vi "1D sweep iteration instruction generator (SubVI).vi"(6 "Maximum value B [µT]":dbl, 7 "Minimum value B [µT]":dbl, 9 "Number of steps":dbl, 10 "Current iteration":i32, 11 "Direction field sweep":string) -> (3 "Current [µT]":dbl, 4 "Magnetic field strength":dbl, 5 "String":string)   [LabVIEW 2018]
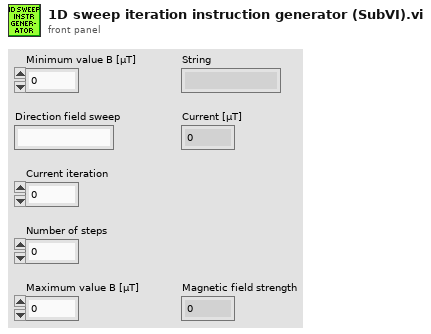
[diagram p1: front panel]
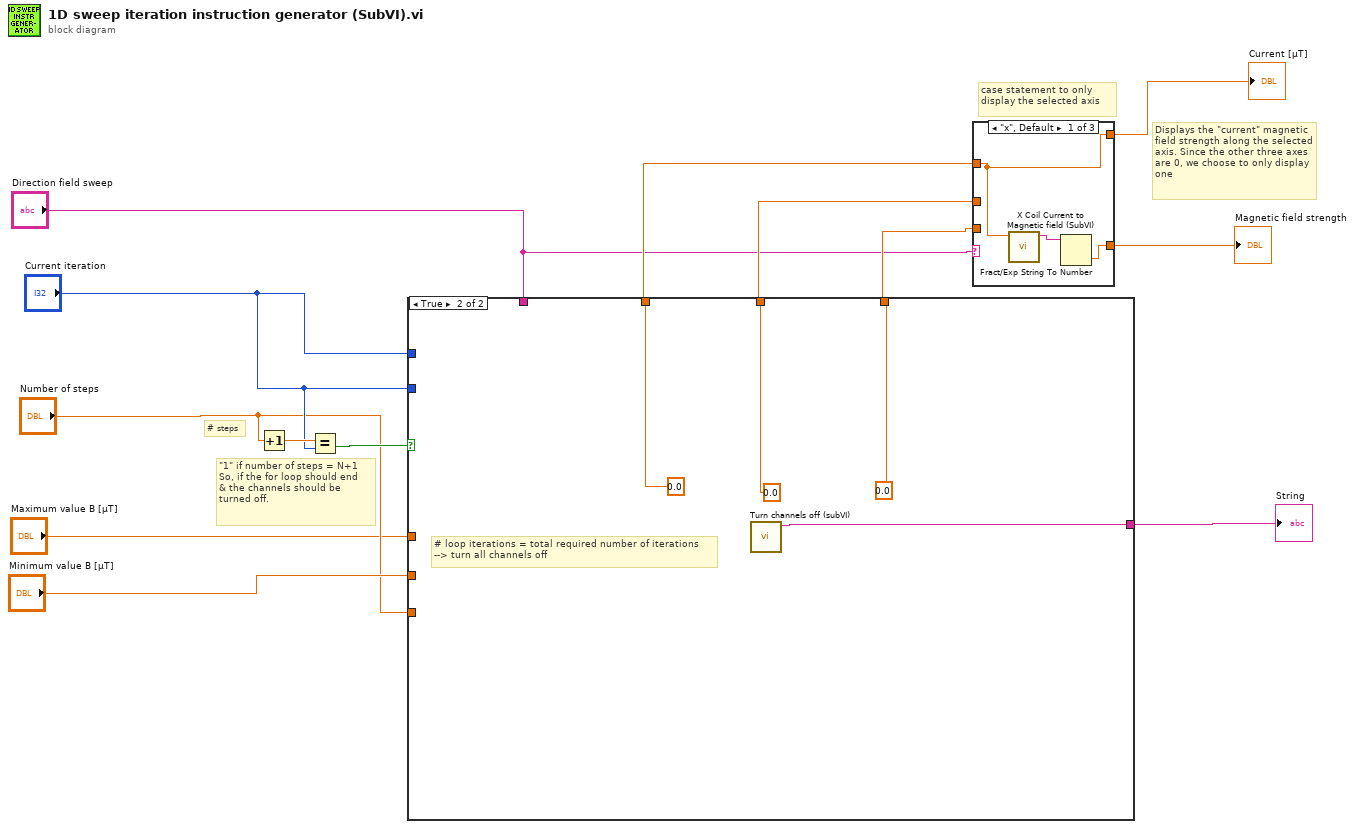
[diagram p0: block diagram]
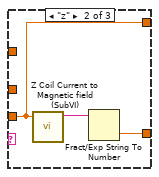
[diagram p2: hidden frame]
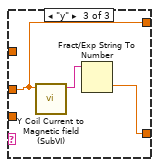
[diagram p3: hidden frame]
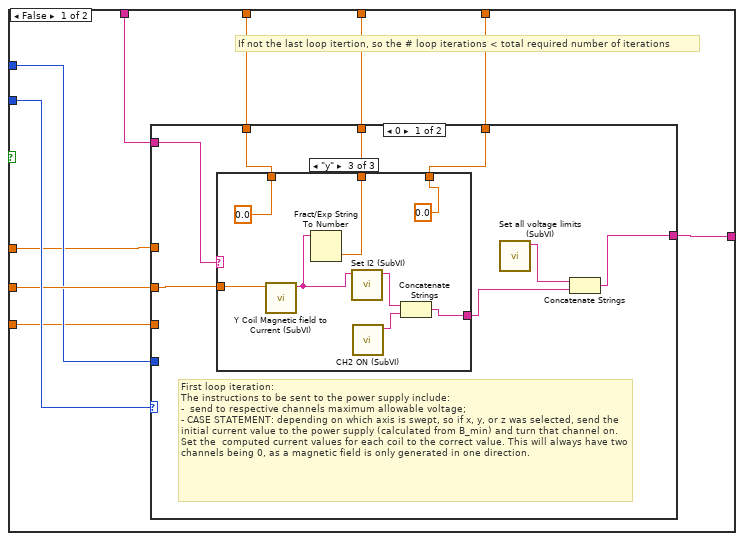
[diagram p4: hidden frame]
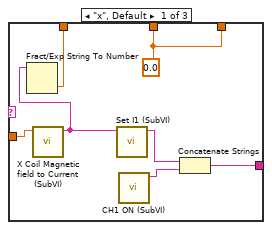
[diagram p5: hidden frame]
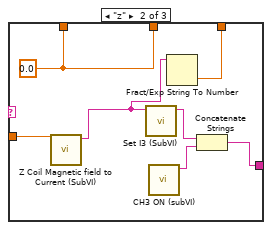
[diagram p6: hidden frame]
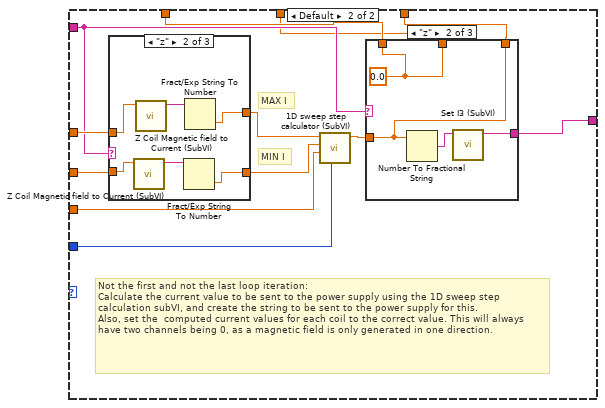
[diagram p7: hidden frame]
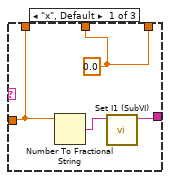
[diagram p8: hidden frame]
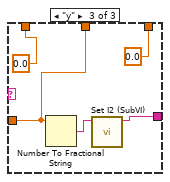
[diagram p9: hidden frame]
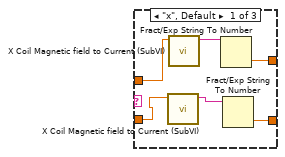
[diagram p10: hidden frame]
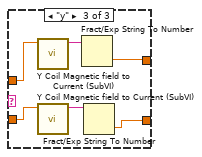
[diagram p11: hidden frame]
diagram:
  # "case statement to only display the selected axis"
  # "Displays the \"current\" magnetic field strength along the selected axis. Since the other three axes are 0, we choose to only display  one"
  # "\"1\" if number of steps = N+1\nSo, if the for loop should end \n& the channels should be \nturned off."
  # "# steps"
  n1 = Increment(x="Number of steps") -> (x+1=w8:dbl)
  n2 = Equal?(x=w8, y="Current iteration") -> (x = y?=w4:bool)
  n3 = case shown="True" w4 {
    tunnel: [w15 0.0 ("Magnetic field x [µT]")] -> w10
    tunnel: [w17 0.0 ("Magnetic field y [µT]")] -> w11
    tunnel: [w16 0.0 ("Magnetic field z [µT]")] -> w12
    tunnel: "Current iteration" -> [w23 _]
    tunnel: "Direction field sweep" -> [w22 _]
    tunnel: "Minimum value B [µT]" -> [w21 _]
    tunnel: "Current iteration" -> [w20 _]
    tunnel: "Number of steps" -> [w19 _]
    tunnel: "Maximum value B [µT]" -> [w18 _]
    tunnel: [w14 w97] -> w6
    frame False {
      # "If not the last loop itertion, so the # loop iterations < total required number of iterations"
      n4 = case shown="0" w23 {
        tunnel: w22 -> [w30 w59]
        tunnel: w21 -> [w31 w65]
        tunnel: w20 -> [_ w60]
        tunnel: w19 -> [_ w61]
        tunnel: w18 -> [_ w64]
        tunnel: [w26 w56] -> w15
        tunnel: [w25 w54] -> w17
        tunnel: [w24 w55] -> w16
        tunnel: [w27 w58] -> w14
        frame 0 {
          # "First loop iteration: \nThe instructions to be sent to the power supply include:\n-  send to respective channels maximum allowable voltage;\n- CASE STATEMENT: depending on which axis is swept, so if x, y, or z was selected, send the initial current value to the power supply (calculated from B_min) and turn that channel on.\nSet the  computed current values for each coil to the correct value. This will always have two channels being 0, as a magnetic field is only generated in one direction."
          n5 = case shown="\"y\"" w30 {
            tunnel: w31 -> [w38 w45 w53]
            tunnel: [w35 w44 w48] -> w29
            tunnel: [w33 w41 0.0 ("Magnetic field y [µT]")] -> w26
            tunnel: [w32 w41 w52] -> w25
            tunnel: [w32 w40 0.0 ("Magnetic field y [µT]")] -> w24
            frame "x", Default {
              w32 = 0.0 ("Magnetic field y [µT]")
              n6 = call "X Coil Magnetic field to Current (SubVI).vi"("Magnetic field [µT]"=w38) -> ("Current X"=w34:string)  [unwired: 10 in]
              n7 = Fract/Exp String To Number(string=w34) -> (number=w33:dbl)  [unwired: 3 in, 1 out]
              n8 = call "Set I1 (SubVI).vi"("Current X"=w34) -> ("String instruction"=w36:string)  [unwired: 10 in]
              n9 = call "CH1 ON (SubVI).vi"() -> ("String"=w37:string)  [unwired: 11 in]
              n10 = Concatenate Strings(w36, w37) -> (w35:string)
            }
            frame "z" {
              w41 = 0.0 ("Magnetic field y [µT]")
              n11 = call "Z Coil Magnetic field to Current (SubVI).vi"("Magnetic field [µT]"=w45) -> ("Current Z"=w39:string)  [unwired: 10 in]
              n12 = call "Set I3 (SubVI).vi"("Current Z"=w39) -> ("String"=w43:string)  [unwired: 10 in]
              n13 = call "CH3 ON (subVI).vi"() -> ("String"=w42:string)  [unwired: 11 in]
              n14 = Fract/Exp String To Number(string=w39) -> (number=w40:dbl)  [unwired: 3 in, 1 out]
              n15 = Concatenate Strings(w43, w42) -> (w44:string)
            }
            frame "y" {
              n16 = call "Y Coil Magnetic field to Current (SubVI).vi"("Magnetic field [µT]"=w53) -> ("Current Y"=w51:string)  [unwired: 10 in]
              n17 = Fract/Exp String To Number(string=w51) -> (number=w52:dbl)  [unwired: 3 in, 1 out]
              n18 = call "Set I2 (SubVI).vi"("Current Y"=w51) -> ("String"=w49:string)  [unwired: 10 in]
              n19 = call "CH2 ON (SubVI).vi"() -> ("String"=w50:string)  [unwired: 11 in]
              n20 = Concatenate Strings(w49, w50) -> (w48:string)
            }
          }
          n21 = call "Set all voltage limits (SubVI).vi"() -> ("String"=w28:string)  [unwired: 11 in]
          n22 = Concatenate Strings(w28, w29) -> (w27:string)
        }
        frame Default {
          # "Not the first and not the last loop iteration: \nCalculate the current value to be sent to the power supply using the 1D sweep step calculation subVI, and create the string to be sent to the power supply for this.  \nAlso, set the  computed current values for each coil to the correct value. This will always have two channels being 0, as a magnetic field is only generated in one direction."
          # "MIN I"
          # "MAX I"
          n23 = case shown="\"z\"" w59 {
            tunnel: w65 -> [w84 w90 w96]
            tunnel: w64 -> [w83 w87 w93]
            tunnel: [w80 w85 w91] -> w63
            tunnel: [w79 w88 w94] -> w62
            frame "x", Default {
              n24 = call "X Coil Magnetic field to Current (SubVI).vi"("Magnetic field [µT]"=w84) -> ("Current X"=w81:string)  [unwired: 10 in]
              n25 = call "X Coil Magnetic field to Current (SubVI).vi"("Magnetic field [µT]"=w83) -> ("Current X"=w82:string)  [unwired: 10 in]
              n26 = Fract/Exp String To Number(string=w82) -> (number=w80:dbl)  [unwired: 3 in, 1 out]
              n27 = Fract/Exp String To Number(string=w81) -> (number=w79:dbl)  [unwired: 3 in, 1 out]
            }
            frame "z" {
              n28 = call "Z Coil Magnetic field to Current (SubVI).vi"("Magnetic field [µT]"=w90) -> ("Current Z"=w89:string)  [unwired: 10 in]
              n29 = call "Z Coil Magnetic field to Current (SubVI).vi"("Magnetic field [µT]"=w87) -> ("Current Z"=w86:string)  [unwired: 10 in]
              n30 = Fract/Exp String To Number(string=w89) -> (number=w88:dbl)  [unwired: 3 in, 1 out]
              n31 = Fract/Exp String To Number(string=w86) -> (number=w85:dbl)  [unwired: 3 in, 1 out]
            }
            frame "y" {
              n32 = call "Y Coil Magnetic field to Current (SubVI).vi"("Magnetic field [µT]"=w93) -> ("Current Y"=w92:string)  [unwired: 10 in]
              n33 = call "Y Coil Magnetic field to Current (SubVI).vi"("Magnetic field [µT]"=w96) -> ("Current Y"=w95:string)  [unwired: 10 in]
              n34 = Fract/Exp String To Number(string=w92) -> (number=w91:dbl)  [unwired: 3 in, 1 out]
              n35 = Fract/Exp String To Number(string=w95) -> (number=w94:dbl)  [unwired: 3 in, 1 out]
            }
          }
          n36 = call "1D sweep step calculator (SubVI).vi"("Iteration"=w60, "Number of steps"=w61, "Minimum current"=w62, "Maximum current"=w63) -> ("Current at this iteration"=w57:dbl)  [unwired: 7 in]
          n37 = case shown="\"z\"" w59 {
            tunnel: [w69 w73 w78] -> w58
            tunnel: w57 -> [w66 w70 w74]
            tunnel: [w66 w72 0.0 ("Magnetic field y [µT]")] -> w56
            tunnel: [w68 w70 0.0 ("Magnetic field y [µT]")] -> w55
            tunnel: [w68 w72 w74] -> w54
            frame "x", Default {
              w68 = 0.0 ("Magnetic field y [µT]")
              n38 = Number To Fractional String(number=w66) -> (F-format string=w67:string)  [unwired: 3 in]
              n39 = call "Set I1 (SubVI).vi"("Current X"=w67) -> ("String instruction"=w69:string)  [unwired: 10 in]
            }
            frame "z" {
              w72 = 0.0 ("Magnetic field y [µT]")
              n40 = Number To Fractional String(number=w70) -> (F-format string=w71:string)  [unwired: 3 in]
              n41 = call "Set I3 (SubVI).vi"("Current Z"=w71) -> ("String"=w73:string)  [unwired: 10 in]
            }
            frame "y" {
              n42 = Number To Fractional String(number=w74) -> (F-format string=w77:string)  [unwired: 3 in]
              n43 = call "Set I2 (SubVI).vi"("Current Y"=w77) -> ("String"=w78:string)  [unwired: 10 in]
            }
          }
        }
      }
    }
    frame True {
      # "# loop iterations = total required number of iterations\n--> turn all channels off"
      n44 = call "Turn channels off (subVI).vi"() -> ("String"=w97:string)  [unwired: 11 in]
    }
  }
  "String" <- w6
  n45 = case shown="\"x\", Default" "Direction field sweep" {
    tunnel: w10 -> [w101 _ _]
    tunnel: w11 -> [_ _ w107]
    tunnel: w12 -> [_ w104 _]
    tunnel: [w103 w105 w109] -> w13
    tunnel: [w101 w104 w107] -> w1
    frame "x", Default {
      n46 = call "X Coil Current to Magnetic field (SubVI).vi"("Current X"=w101) -> ("Magnetic field X [µT]"=w102:string)  [unwired: 10 in]
      n47 = Fract/Exp String To Number(string=w102) -> (number=w103:dbl)  [unwired: 3 in, 1 out]
    }
    frame "z" {
      n48 = call "Z Coil Current to Magnetic field (SubVI).vi"("Current Z"=w104) -> ("Magnetic field Z [µT]"=w106:string)  [unwired: 10 in]
      n49 = Fract/Exp String To Number(string=w106) -> (number=w105:dbl)  [unwired: 3 in, 1 out]
    }
    frame "y" {
      n50 = call "Y Coil Current to Magnetic field (SubVI).vi"("Current Y"=w107) -> ("Magnetic field Y [µT]"=w108:string)  [unwired: 10 in]
      n51 = Fract/Exp String To Number(string=w108) -> (number=w109:dbl)  [unwired: 3 in, 1 out]
    }
  }
  "Magnetic field strength" <- w13
  "Current [µT]" <- w1
